vi "34461ATrigger.vi"() -> ()   [LabVIEW 2014]
uses:
  <instrlib>/Agilent 3446X Series/Public/Data/Read (Single Point).vi
  <instrlib>/Agilent 3446X Series/Agilent 3446X Series.lvlib
panel:
  in  "Manual Range":dbl=10.0
  out "波形图表":dbl[](graph)
  in  "Sample Period(ms)":dbl=100.0
  out "已采样数量":dbl
  in  "Data Collection Switch":bool
  in  "Aperture Time":sgl(ring)=1.0 items=["100"=100, "10"=10, "1"=1, "0.2"=0.2, "0.02"=0.02]
  in  "Auto Zero":enum16{"Off", "On"}(ring)=enum."On"
  in  "VISA resource name":refnum<visa-resource-name>
  in  "Auto Range":bool=TRUE
  in  "Absolute Resolution":dbl=1e-06
  in  "Measurement Function":i32(ring)=10 items=["Continuity", "Current AC", "Current DC", "Diode", "Frequency", "Resistance 4-wire", "Period", "Resistance 2-wire", "Temperature", "Voltage AC", "Voltage DC", "Voltage DC Ratio"]
  in  "路径":path=path "data"
  # "Note：before running the program ,open the Data Collection Switch .Use the Data Collection Switch to stop the program."
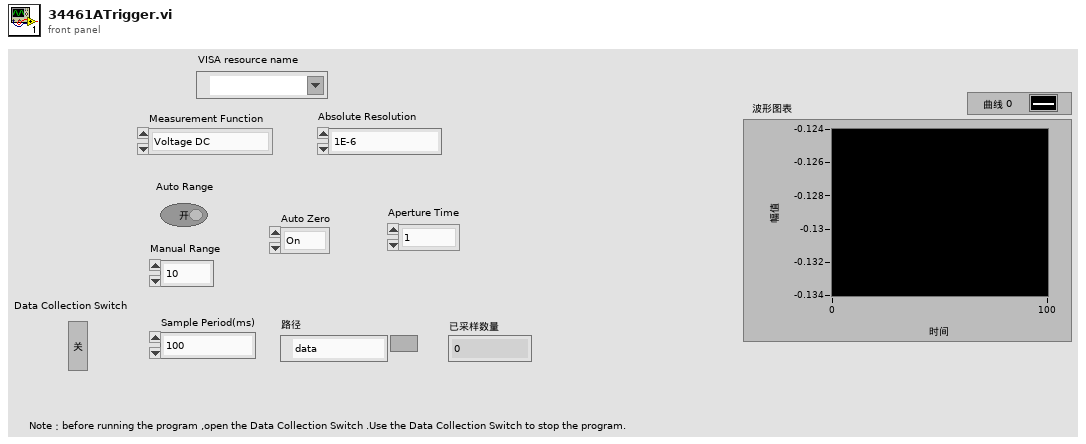
[diagram p1: front panel]
types:
  T1 = enum16{"open", "open or create", "create or replace", "create", "open (read-only)"}
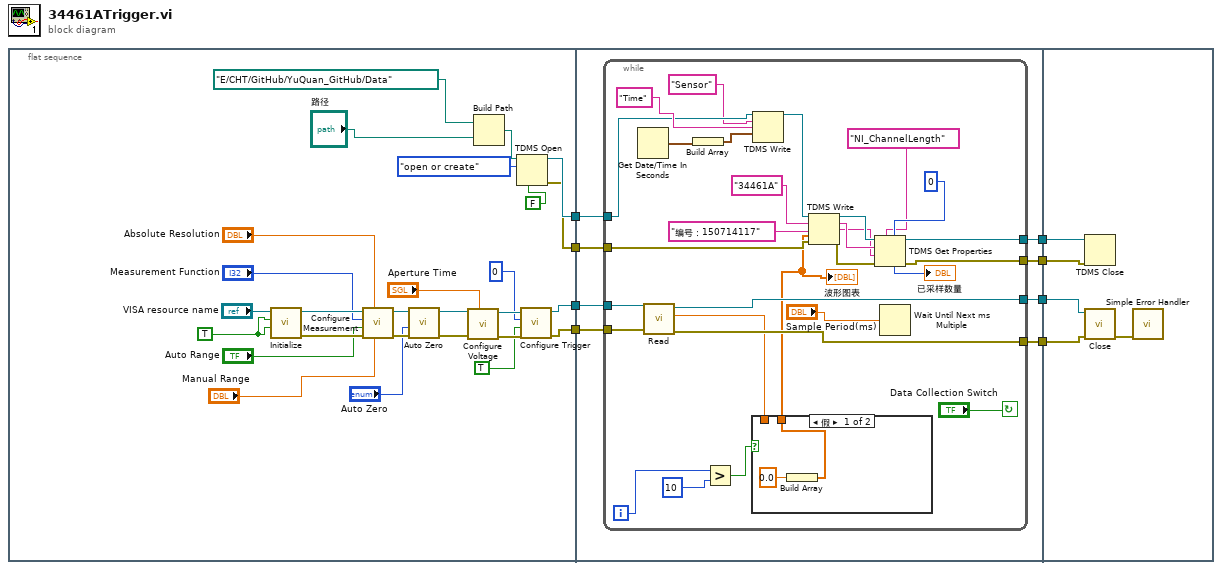
[diagram p0: block diagram]
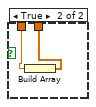
[diagram p2: hidden frame]
diagram:
  n1 = flat-sequence {
    tunnel: [w10] -> w8
    tunnel: [w9] -> w7
    tunnel: [w23] -> w6
    tunnel: [w22] -> w2
    tunnel: w8 -> [w42]
    tunnel: w7 -> [w41]
    tunnel: w6 -> [w43]
    tunnel: [w40] -> w5
    tunnel: [w39] -> w4
    tunnel: [w38] -> w3
    tunnel: w2 -> [w37]
    tunnel: [w36] -> w1
    tunnel: w5 -> [w80]
    tunnel: w4 -> [w79]
    tunnel: w3 -> [w78]
    tunnel: w1 -> [w77]
    frame #0 {
      w21 = TRUE
      n2 = call <instrlib>:"Initialize.vi"("Reset (True)"=w21, "ID Query (True)"=w21, "VISA resource name"="VISA resource name") -> ("error out"=w30:errorcluster, "VISA resource name out"=w31:refnum<visa-resource-name>)  [unwired: 2 in, 5 out]
      n3 = call <instrlib>:"Configure Measurement.vi"("Manual Range (1)"="Manual Range", "Absolute Resolution (1E-6)"="Absolute Resolution", "error in (no error)"=w30, "Auto Range (T: Enable)"="Auto Range", "Measurement Function (10: Voltage DC)"="Measurement Function", "VISA resource name"=w31) -> ("error out"=w25:errorcluster, "VISA resource name out"=w24:refnum<visa-resource-name>)  [unwired: 4 out]
      n4 = call <instrlib>:"Auto Zero.vi"("error in (no error)"=w25, "Auto Zero (1: Enable)"="Auto Zero", "VISA resource name"=w24) -> ("error out"=w17:errorcluster, "VISA resource name out"=w18:refnum<visa-resource-name>)  [unwired: 7 in]
      n5 = call <instrlib>:"Configure Voltage.vi"("Voltage Integration Time (10: 10)"="Aperture Time", "error in (no error)"=w17, "VISA resource name"=w18) -> ("error out"=w13:errorcluster, "VISA resource name out"=w14:refnum<visa-resource-name>)  [unwired: 7 in]
      n6 = Build Path(base path=path "E:/CHT/GitHub/YuQuan_GitHub/Data", name or relative path="路径") -> (appended path=w35:path)
      n7 = TDMS Open(6:FALSE ("disable buffering (T)"), 10:T1."open or create" ("operation"), 11:w35) -> (0:w22:errorcluster, 3:w23:refnum<k34>)  [unwired: 4 in]
      n8 = call <instrlib>:"Configure Trigger.vi"("error in (no error)"=w13, "Auto Delay (T:Enable)"=TRUE, "Trigger Source (0: Immediate)"=0, "VISA resource name"=w14) -> ("error out"=w9:errorcluster, "VISA resource name out"=w10:refnum<visa-resource-name>)  [unwired: 6 in]
    }
    frame #1 {
      n9 = while {
        tunnel: w43 -> [w54]
        tunnel: w42 -> [w47]
        tunnel: w41 -> [w46]
        tunnel: [w64] -> w40
        tunnel: [w63] -> w39
        tunnel: [w62] -> w38
        tunnel: w37 -> [w61]
        tunnel: [w59] -> w36
        i -> [w51]
        stop <- "Data Collection Switch" continue-if-true
        n10 = Get Date/Time In Seconds() -> (seconds since 1Jan1904=w57:timestamp)
        n11 = call-poly <instrlib>:"Read.vi"("error in (no error)"=w46, "VISA resource name"=w47) -> ("error out"=w63:errorcluster, "Measurement"=w45:dbl, "VISA resource name out"=w64:refnum<visa-resource-name>)  [unwired: 1 in, 6 out]
        n12 = Build Array(w57) -> (w56:timestamp[])
        n13 = Greater?(x=w51, y=10) -> (0:w49:bool)
        n14 = case shown="假" w49 {
          tunnel: w45 -> [_ w76]
          tunnel: [w73 w75] -> w44
          frame False {
            n15 = Build Array(0.0) -> (w73:dbl[])
          }
          frame True {
            n16 = Build Array(w76) -> (w75:dbl[])
          }
        }
        "波形图表" <- w44
        n17 = TDMS Write(0:w54, 5:"Sensor", 7:"Time", 9:w56) -> (4:w53:refnum<k34>)  [unwired: 2 in, 3 out]
        n18 = TDMS Write(0:w53, 5:"34461A", 7:"编号：150714117", 9:w44, 11:w61) -> (4:w69:refnum<k34>, 6:w68:string, 8:w67:string, 15:w60:errorcluster)  [unwired: 1 in]
        n19 = TDMS Get Properties(5:0, 7:"NI_ChannelLength", 8:w60, 9:w67, 10:w68, 11:w69) -> (0:w59:errorcluster, 3:w62:refnum<k34>, 4:→"已采样数量":i32)  [unwired: 3 out]
        n20 = Wait Until Next ms Multiple(millisecond multiple="Sample Period(ms)") -> ()  [unwired: 1 out]
      }
    }
    frame #2 {
      n21 = TDMS Close(8:w77, 11:w78) -> ()  [unwired: 2 out]
      n22 = call <instrlib>:"Close.vi"("error in (no error)"=w79, "VISA resource name"=w80) -> ("error out"=w81:errorcluster)  [unwired: 9 out]
      n23 = call <vilib>:"Simple Error Handler.vi"("error in (no error)"=w81) -> ()  [unwired: 1 in, 8 out]
    }
  }
